vi "GetSRs.vi"(7 "LabVIEW Web Service Request":refnum<class "Web Request.lvclass">) -> (3 "SRListOut":T1 {"SR#" format="%#_10g"})   [LabVIEW 2017]
uses:
  <vilib>/wsapi/Web Request.lvclass
  ServerLib/TypeDefs/SR List.ctl
  ServerLib/TypeDefs/SR Data.ctl
  ServerLib/SubLibs/WebServiceCommunication/WebServiceFGVcommands.ctl
  ServerLib/SubLibs/WebServiceCommunication/WebServiceCommunication.lvlib
  ServerLib/SubLibs/ErrorLogger/ErrorLogger.lvlib
  ServerLib/Server.lvlib
panel:
  out "error out":errorcluster
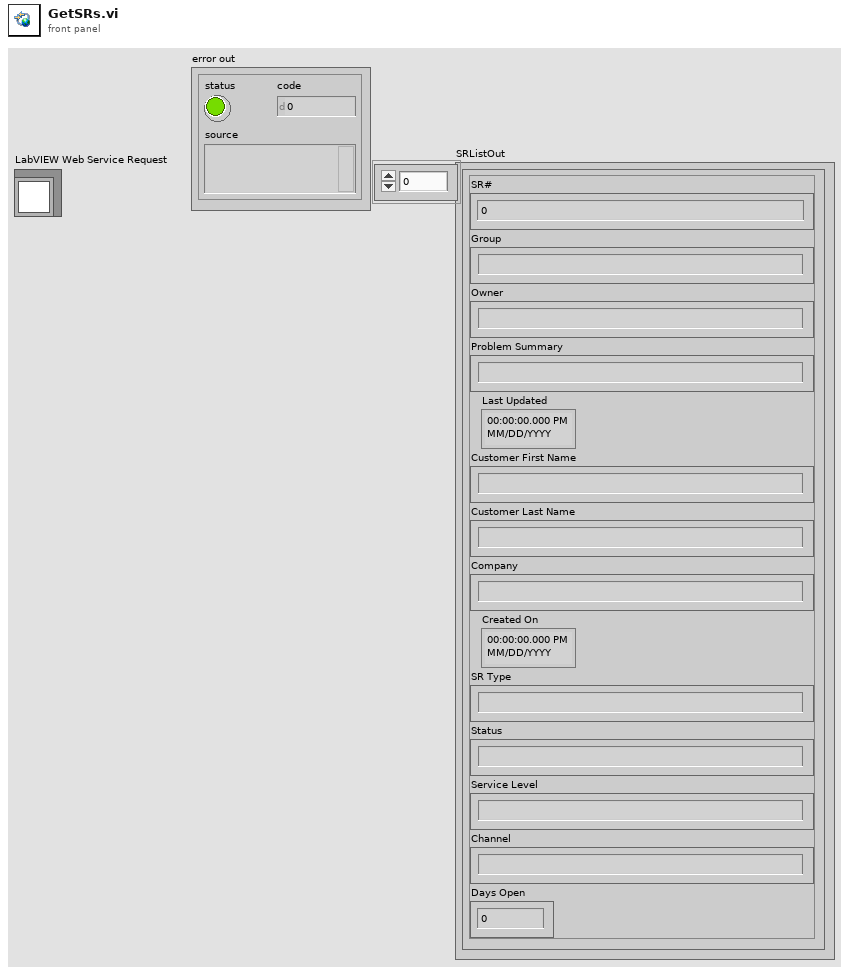
[diagram p1: front panel]
types:
  T1 = typedef "Server.lvlib/SR List.ctl" = T2[]
  T2 = typedef "Server.lvlib/SR Data.ctl" = cluster{"SR#":dbl, "Group":string, "Owner":string, "Problem Summary":string, "Last Updated":timestamp, "Customer First Name":string, "Customer Last Name":string, "Company":string, "Created On":timestamp, "SR Type":string, "Status":string, "Service Level":string, "Channel":string, "Days Open":dbl}
  T3 = typedef "Server.lvlib/WebServiceCommunication.lvlib/WebServiceFGVcommands.ctl" = enum16{"Init", "Reset", "Heartbeat", "GetSRs", "SetSRs", "CheckClients", "GetClients"}
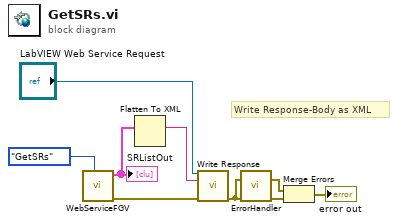
[diagram p0: block diagram]
diagram:
  # "Write Response-Body as XML"
  n1 = call "WebServiceFGV.vi"("CMD"=WebServiceFGVcommands."GetSRs") -> ("error out"=w4:errorcluster, "SRListOut"=w6:T1)  [unwired: 8 in, 1 out]
  "SRListOut" <- w6
  n2 = Flatten To XML(anything=w6) -> (xml string=w5:string)
  n3 = call <vilib>:"Write Response.vi"("LabVIEW Web Service Request"="LabVIEW Web Service Request", "response string"=w5, "error in (no error)"=w4) -> ("error out"=w2:errorcluster)  [unwired: 11 in, 1 out]
  n4 = call "ErrorHandler.vi"("error in (no error)"=w2) -> ("error out"=w3:errorcluster)  [unwired: 10 in]
  n5 = Merge Errors(w2, w3) -> (→"error out":errorcluster)
